vi "RetrieveMeasurementValues&Attributes.vi"(7 "PlotYScale":u32[](array[numeric]), 8 "error in (no error)":errorcluster, 10 "Variant":variant, 11 "WaveformChartReference":refnum<vi>) -> (0 "error out":errorcluster, 1 "Incorrect DataType?":bool, 2 "Array Of Strings":string[](array[string]), 3 "WaveformArrayOut":waveform(dbl)[](array[waveform]))   [LabVIEW 2018, in "Visualization.lvlib" / "VisualizeSensor.lvclass"]
uses:
  VisualizeSensor.lvclass
  Sensor/SensorShared/SiemensDEMMeasurements.ctl
  Sensor/SensorShared/SensorShared.lvlib
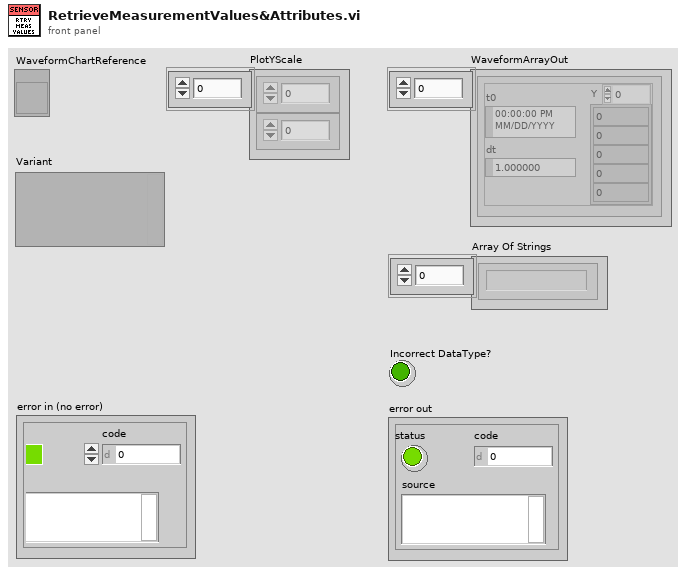
[diagram p1: front panel]
types:
  T1 = typedef "SensorShared.lvlib/SiemensDEMMeasurements.ctl" = cluster{"Array of Waveforms":waveform(dbl)[], "Array of Strings ":string[]}
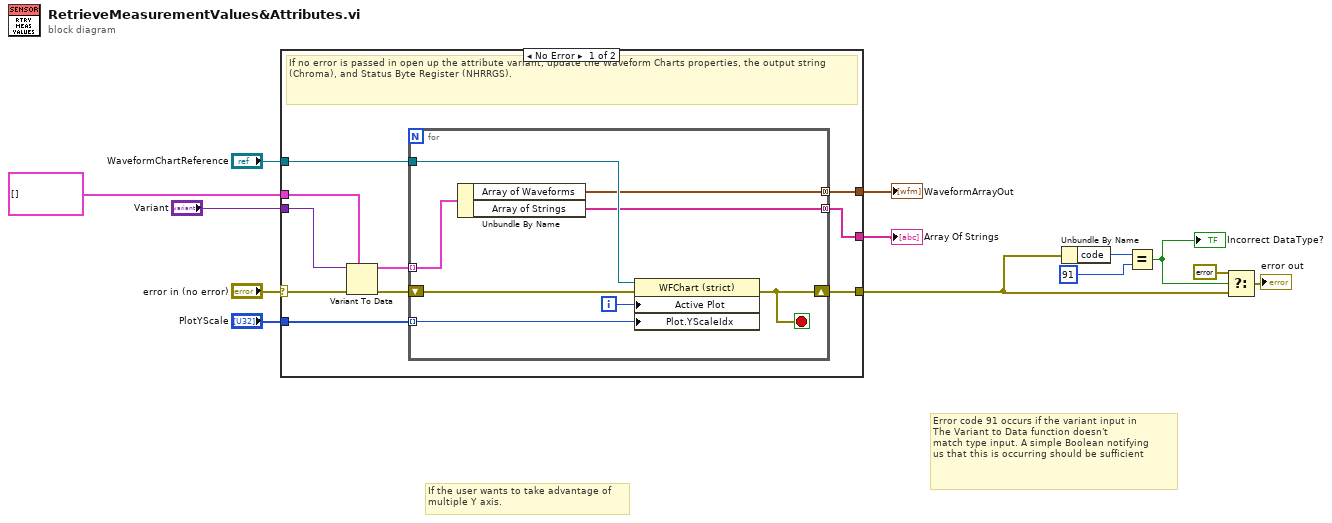
[diagram p0: block diagram]
diagram:
  # "If the user wants to take advantage of \nmultiple Y axis."
  # "Error code 91 occurs if the variant input in \nThe Variant to Data function doesn't \nmatch type input. A simple Boolean notifying \nus that this is occurring should be sufficient"
  n1 = case shown="No Error" "error in (no error)" {
    selector: "error in (no error)" -> [w19 w32]
    tunnel: [w23 w32] -> w5
    tunnel: [w22 _] -> w4
    tunnel: "WaveformChartReference" -> [w20 _]
    tunnel: "PlotYScale" -> [w21 _]
    tunnel: "Variant" -> [w17 _]
    tunnel: T1[] [] -> [w16 _]
    tunnel: [w14 _] -> w1
    frame No Error {
      # "If no error is passed in open up the attribute variant, update the Waveform Charts properties, the output string (Chroma), and Status Byte Register (NHRRGS)."
      n2 = Variant To Data(error in=w19, type=w16, Variant=w17) -> (data=w15:T1[], error out=w18:errorcluster)
      n3 = for {
        shift-right: [w28] -> w23
        shift-left: w18 -> [w27]
        tunnel: [w24] -> w22 mode=concatenating
        tunnel: w20 -> [w30]
        tunnel: w21 -> [w29] mode=indexing
        tunnel: w15 -> [w26] mode=indexing
        tunnel: [w25] -> w14 mode=concatenating
        i -> [w31]
        stop <- w28 stop-if-true
        n4 = Unbundle By Name(w26) -> ("Array of Waveforms"=w24:waveform(dbl)[], "Array of Strings"=w25:string[])
        n5 = property on="Property Node" class="WFChart (strict)"(reference=w30, error in=w27, "Active Plot"=w31, "Plot.YScaleIdx"=w29) -> (error out=w28:errorcluster)  [unwired: 1 out]
      }
    }
    frame Error {
    }
  }
  "WaveformArrayOut" <- w4
  "Array Of Strings" <- w1
  n6 = Unbundle By Name(w5) -> ("code"=w10:i32)
  n7 = Equal?(x=w10, y=91) -> (x = y?=w8:bool)
  "Incorrect DataType?" <- w8
  n8 = Select(t=errorcluster {"status"=FALSE, "code"=0, "source"=""} ("error IO"), s=w8, f=w5) -> (s? t:f=→"error out":errorcluster)
